vi "Save TextConstant to md.vi"(8 "Error In (No Error) 2":errorcluster, 10 "Array 2":cluster{refnum<vi>, "Text":string}[](array[cluster]), 11 "Path 2":path) -> (0 "Error Out 2":errorcluster)   [LabVIEW 2017]
uses:
  _tool/_file/csm-file-support.lvlib
  Communicable State Machine.lvlib
  _Shared/CSM Shared.lvlib
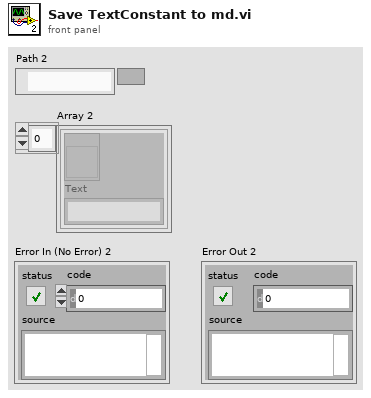
[diagram p1: front panel]
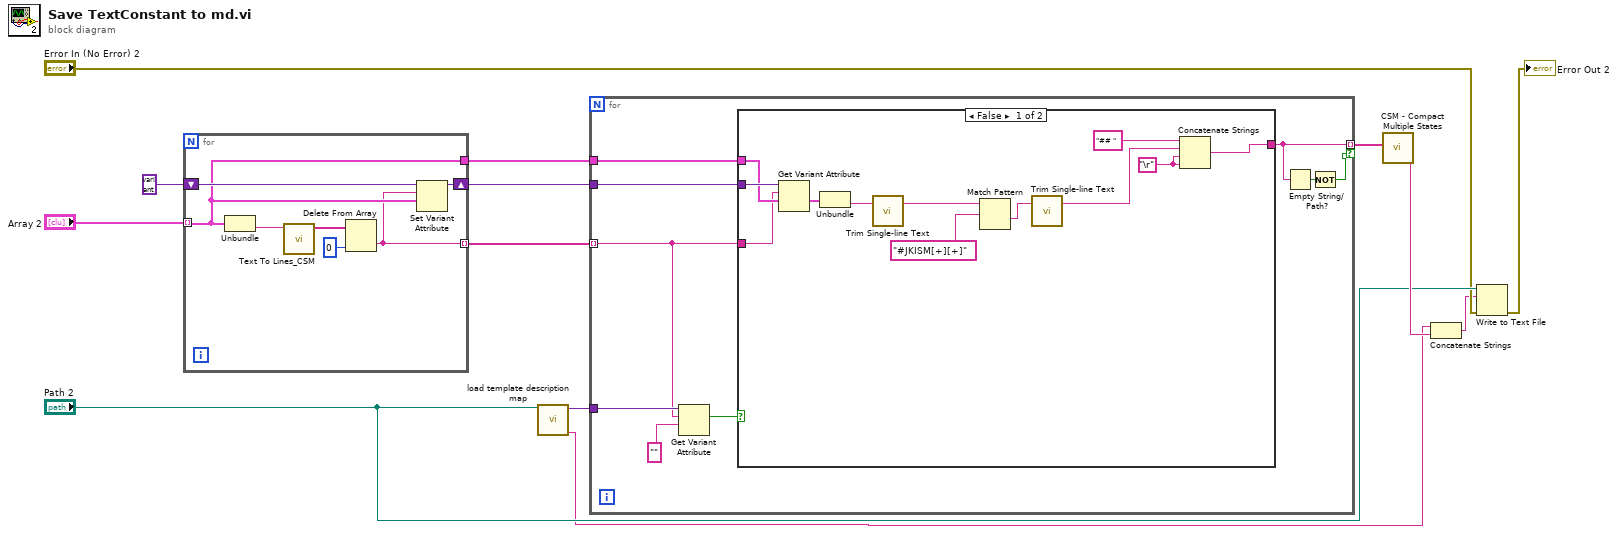
[diagram p0: block diagram]
diagram:
  n1 = for {
    tunnel: "Array 2" -> [w15] mode=indexing
    shift-right: [w17] -> w10
    shift-left: variant -> [w16]
    tunnel: [w15] -> w9
    tunnel: [w14] -> w8 mode=indexing
    n2 = Unbundle(w15) -> ("Text"=w20:string)  [unwired: 1 out]
    n3 = call "Text To Lines_CSM.vi"("String"=w20) -> ("Lines"=w18:string[])  [unwired: 9 in, 1 out]
    n4 = Delete From Array(array=w18, index=0) -> (deleted portion=w14:string)  [unwired: 1 in, 1 out]
    n5 = Set Variant Attribute(Variant=w16, name=w14, value=w15) -> (Variant out=w17:variant)  [unwired: 1 in, 2 out]
  }
  n6 = call "load template description map.vi"("Path"="Path 2") -> ("Text"=w1:string, "Variant"=w13:variant)  [unwired: 8 in, 1 out]
  n7 = for {
    tunnel: w10 -> [w28]
    tunnel: w9 -> [w27]
    tunnel: w13 -> [w29]
    tunnel: w8 -> [w24] mode=indexing
    tunnel: [w23] -> w7 mode=indexing if=w21
    n8 = Get Variant Attribute(Variant=w29, name=w24, default value (empty Variant)="" ("deleted portion")) -> (found=w25:bool)  [unwired: 1 in, 3 out]
    n9 = case shown="False" w25 {
      tunnel: w28 -> [w41 _]
      tunnel: w27 -> [w40 _]
      tunnel: w24 -> [w38 _]
      tunnel: [w36 _] -> w23
      frame False {
        w35 = "\r"
        n10 = Get Variant Attribute(Variant=w41, name=w38, default value (empty Variant)=w40) -> (value=w39:cluster{refnum<vi>, "Text":string})  [unwired: 1 in, 3 out]
        n11 = Unbundle(w39) -> ("Text"=w34:string)  [unwired: 1 out]
        n12 = call "Trim Single-line Text.vi"("single-line text"=w34) -> ("trimed text"=w32:string)  [unwired: 2 in]
        n13 = Match Pattern(string=w32, regular expression="#JKISM[+][+]") -> (after substring=w30:string)  [unwired: 1 in, 3 out]
        n14 = call "Trim Single-line Text.vi"("single-line text"=w30) -> ("trimed text"=w31:string)  [unwired: 2 in]
        n15 = Concatenate Strings("## " ("string"), w31, w35, w35) -> (w36:string)
      }
      frame True {
      }
    }
    n16 = Empty String/Path?(string/path=w23) -> (empty?=w22:bool)
    n17 = Not(x=w22) -> (.not. x?=w21:bool)
  }
  n18 = call "CSM - Compact Multiple States.vi"("Multiple States"=w7) -> ("States"=w6:string)  [unwired: 9 in]
  n19 = Concatenate Strings(w1, w6) -> (w2:string)
  n20 = Write to Text File(file (use dialog)="Path 2", text=w2, error in="Error In (No Error) 2") -> (error out=→"Error Out 2":errorcluster)  [unwired: 1 in, 2 out]
